vi "DepthToVolume.vi"(8 "error in (no error)":errorcluster, 9 "Objects In":T2[](array[typedef]) {"Nb Holes" format="%.2f"; "Aspect Ratio" format="%.2f"; "Orientation" format="%.2f"; "Area" format="%.2f"; "Bounding Box"."Y Top" format="%.2f"; "Bounding Box"."X Left" format="%.2f"; "Object Center"."Y" format="%.2f"; "Object Center"."X" format="%.2f"}, 10 "Trigger 1/L":bool, 11 "Depth In":T1) -> (0 "error out":errorcluster, 2 "Volume 1/L":fxp<+,8,0>, 4 "Clear":bool)   [LabVIEW 2015]
uses:
  TypeDefs Host/Object Info.ctl
  <vilib>/vision/Image Controls.llb/IMAQ Image.ctl
  TypeDefs Host/Open Audio FGV Enum.ctl
panel:
  out "Volume R":fxp<+,8,0>
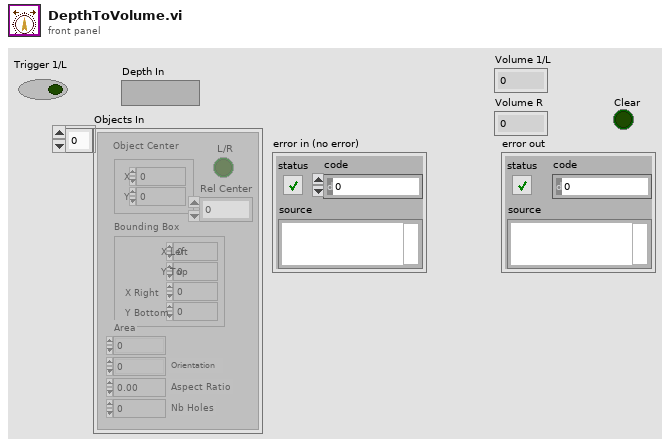
[diagram p1: front panel]
types:
  T1 = typedef "IMAQ Image.ctl" = refnum<image>
  T2 = typedef "Object Info.ctl" = cluster{"Object Center":cluster{"X":u16, "Y":u16}, "Bounding Box":cluster{"X Left":u16, "Y Top":u16, "X Right":u16, "Y Bottom":u16}, "Area":u16, "Orientation":u16, "Aspect Ratio":sgl, "Nb Holes":u16, "L/R":bool, "Rel Center":u16}
  T3 = typedef "Open Audio FGV Enum.ctl" = enum16{"Get", "Set"}
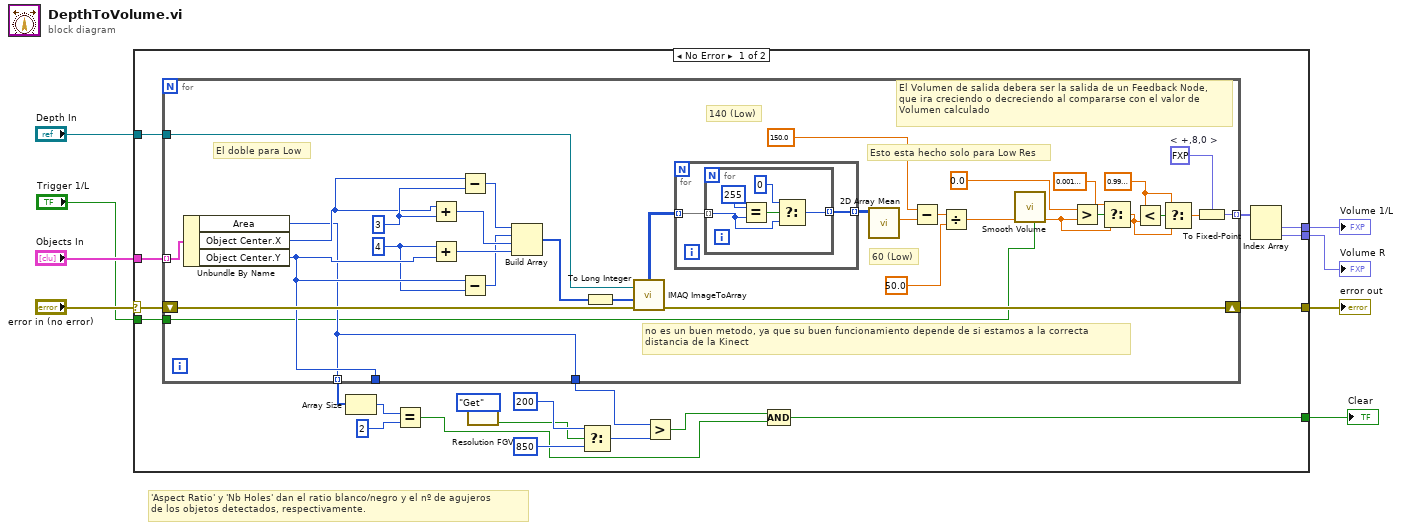
[diagram p0: block diagram]
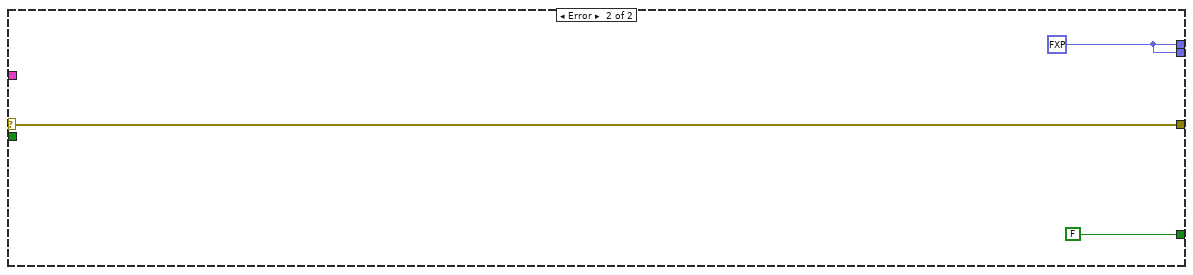
[diagram p2: hidden frame]
diagram:
  # "'Aspect Ratio' y 'Nb Holes' dan el ratio blanco/negro y el nº de agujeros\nde los objetos detectados, respectivamente."
  n1 = case shown="No Error" "error in (no error)" {
    selector: "error in (no error)" -> [w23 w71]
    tunnel: [w28 w71] -> w8
    tunnel: "Objects In" -> [w27 _]
    tunnel: "Depth In" -> [w22 _]
    tunnel: [w11 w69] -> w3
    tunnel: [w24 FALSE] -> w4
    tunnel: [w10 w69] -> w2
    tunnel: "Trigger 1/L" -> [w9 _]
    frame No Error {
      n2 = for {
        tunnel: w22 -> [w60]
        tunnel: w27 -> [w59] mode=indexing
        shift-right: [w61] -> w28
        shift-left: w23 -> [w58]
        tunnel: [w32] -> w26 mode=indexing
        tunnel: [w32] -> w17
        tunnel: [w34] -> w12 mode=indexing
        tunnel: [w57] -> _
        tunnel: w9 -> [w29]
        w35 = fxp<+,8,0> 0.0  # < +,8,0 >
        w37 = sgl 0.99 ("y")
        w50 = u16 4
        w53 = u16 3
        # "El doble para Low"
        # "60 (Low)"
        # "140 (Low)"
        # "El Volumen de salida debera ser la salida de un Feedback Node,\nque ira creciendo o decreciendo al compararse con el valor de \nVolumen calculado"
        # "Esto esta hecho solo para Low Res"
        # "no es un buen metodo, ya que su buen funcionamiento depende de si estamos a la correcta\ndistancia de la Kinect"
        n3 = Unbundle By Name(w59) -> ("Area"=w32:u16, "Object Center.X"=w44:u16, "Object Center.Y"=w57:u16)
        n4 = Add(x=w44, y=w53) -> (x+y=w55:u16)
        n5 = Add(x=w50, y=w57) -> (x+y=w52:u16)
        n6 = Subtract(x=w44, y=w53) -> (x-y=w54:u16)
        n7 = Subtract(x=w57, y=w50) -> (x-y=w51:u16)
        n8 = Build Array(w54, w51, w55, w52) -> (w56:u16[])
        n9 = To Long Integer(number=w56) -> (32bit integer=w33:i32[])
        n10 = call "IMAQ ImageToArray"("error in (no error)"=w58, "Optional Rectangle"=w33, "Image"=w60) -> ("error out"=w61:errorcluster, "Image Pixels (U8)"=w49:u8[][])  [unwired: 1 in, 3 out]
        n11 = for {
          tunnel: w49 -> [w63] mode=indexing
          tunnel: [w62] -> w48 mode=indexing
          n12 = for {
            tunnel: w63 -> [w65] mode=indexing
            tunnel: [w64] -> w62 mode=indexing
            n13 = Equal?(x=u8 255, y=w65) -> (x = y?=w67:bool)
            n14 = Select(t=u8 0 ("x"), s=w67, f=w65) -> (s? t:f=w64:u8)
          }
        }
        n15 = call "2D Array Mean.vi"("Image Pixels (U8)"=w48) -> ("mean"=w43:dbl)  [unwired: 10 in]
        n16 = Subtract(x=150.0 ("y"), y=w43) -> (x-y=w46:dbl)
        n17 = Divide(x=w46, y=50.0 ("y 2")) -> (x/y=w31:dbl)
        n18 = call "Smooth Volume.vi"("Trigger"=w29, "Volume In"=w31) -> ("Volume Out"=w30:sgl)  [unwired: 9 in]
        n19 = Greater?(x=sgl 0.0 ("y"), y=w30) -> (0:w41:bool)
        n20 = Select(t=sgl 0.001 ("Volume Left"), s=w41, f=w30) -> (s? t:f=w38:sgl)
        n21 = Less?(x=w37, y=w38) -> (x < y?=w39:bool)
        n22 = Select(t=w37, s=w39, f=w38) -> (s? t:f=w36:sgl)
        n23 = To Fixed-Point(fixed-point type=w35, number=w36) -> (fixed-point=w34:fxp<+,8,0>)
      }
      n24 = Array Size(array=w26) -> (size(s)=w13:i32)
      n25 = Equal?(x=w13, y=2) -> (x = y?=w14:bool)
      n26 = call "Resolution FGV.vi"("Command"=Open_Audio_FGV_Enum."Get") -> ("L/T?"=w15:bool)  [unwired: 10 in]
      n27 = Select(t=u16 200 ("x"), s=w15, f=u16 850 ("x")) -> (s? t:f=w16:u16)
      n28 = Greater?(x=w17, y=w16) -> (0:w18:bool)
      n29 = Compound Arithmetic op=AND(w18, w14) -> (w24:bool)
      n30 = Index Array(array=w12) -> (element #1=w11:fxp<+,8,0>, element #2=w10:fxp<+,8,0>)  [unwired: 2 in]
    }
    frame Error {
      w69 = fxp<+,8,0> 0.0 ("< +,8,0 >")
    }
  }
  "error out" <- w8
  "Clear" <- w4
  "Volume 1/L" <- w3
  "Volume R" <- w2
